vi "DAQ DI.vi"(8 "error in":errorcluster, 11 "Alias":string="Relay") -> (0 "error out":errorcluster={"status"=TRUE, "code"=91, "source"="Variant To Data in MIO Wrappers.lvlib:DAQ DI.vi"}, 3 "Bit":bool)   [LabVIEW 2021, in "Wrappers.lvlib"]
uses:
  Wrappers.lvlib
  Load INI/Controls/DAQ_Data.ctl
  <vilib>/DAQmx/read.llb/DAQmx Read (Digital Bool 1Line 1Point).vi
  <vilib>/DAQmx/create/channels.llb/DAQmx Create Channel (DI-Digital Input).vi
  <vilib>/DAQmx/miscellaneous.llb/DAQmx Fill In Error Info.vi
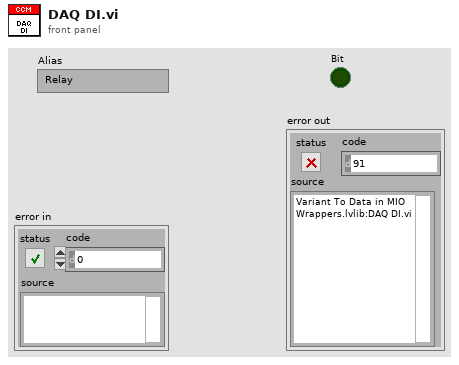
[diagram p1: front panel]
types:
  T1 = typedef "DAQ_Data.ctl" = cluster{"Alias":string, "MUX":string, "Route":string, "Channel":string}
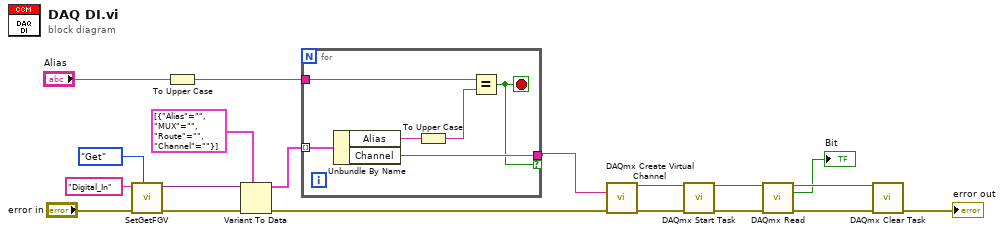
[diagram p0: block diagram]
diagram:
  n1 = call "SetGetFGV.vi"("Method (Get)"=enum16{"Get", "Set"}."Get", "error in"="error in", "FGVname"="Digital_In" ("Name")) -> ("error out"=w11:errorcluster, "Data out"=w10:variant)  [unwired: 7 in]
  n2 = To Upper Case(1:"Alias") -> (0:w3:string)
  n3 = Variant To Data(error in=w11, type=T1[] [{"Alias"="", "MUX"="", "Route"="", "Channel"=""}], Variant=w10) -> (data=w6:T1[], error out=w7:errorcluster)
  n4 = for {
    tunnel: w6 -> [w25] mode=indexing
    tunnel: [w24] -> w4 if=w21
    tunnel: w3 -> [w23]
    stop <- w21 stop-if-true
    n5 = Unbundle By Name(w25) -> ("Alias"=w22:string, "Channel"=w24:string)
    n6 = To Upper Case(1:w22) -> (0:w20:string)
    n7 = Equal?(x=w23, y=w20) -> (x = y?=w21:bool)
  }
  n8 = call-poly <vilib>:"DAQmx Create Virtual Channel.vi"("lines"=w4, "error in"=w7) -> ("task out"=w15:refnum<k21>, "error out"=w16:errorcluster)  [unwired: 12 in]
  n9 = call <vilib>:"DAQmx Start Task.vi"("task/channels in"=w15, "error in"=w16) -> ("task out"=w18:refnum<k21>, "error out"=w17:errorcluster)  [unwired: 12 in]
  n10 = call-poly <vilib>:"DAQmx Read.vi"("task/channels in"=w18, "error in"=w17) -> ("task out"=w14:refnum<k21>, "data"=→"Bit":bool, "error out"=w13:errorcluster)  [unwired: 11 in]
  n11 = call <vilib>:"DAQmx Clear Task.vi"("task in"=w14, "error in"=w13) -> ("error out"=→"error out":errorcluster)  [unwired: 13 in]
